vi "test bindata to typed num array.vi"() -> ()   [LabVIEW 2018, in "LV-Julia_ZMQ-Roundtrip_lib.lvlib"]
uses:
  LV-Julia_ZMQ-Roundtrip_lib.lvlib
  ce04cff8-4bf9-4973-825c-a5c8130598ec.vi
panel:
  out "Num Array out":dbl[][](array[numeric])
  in  "Array type in":dbl[](array[numeric])
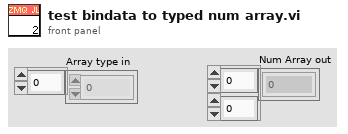
[diagram p1: front panel]
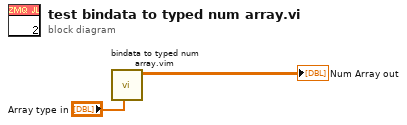
[diagram p0: block diagram]
diagram:
  n1 = call "bindata to typed num array.vim"("Array type in"="Array type in") -> ("Num Array out"=→"Num Array out":dbl[][])  [unwired: 10 in]
